vi "acqWaveform - 副本.vi"(0 "OSC in":refnum<visa-resource-name>, 1 "Points":u32=2000 max=7000, 2 "error in (no error)":errorcluster) -> (3 "OSC out":refnum<visa-resource-name>, 4 "time sequence":dbl[](array[numeric]), 5 "Voltage sequence":dbl[](array[numeric]), 6 "error out":errorcluster)   [LabVIEW 2016]
panel:
  out "XY Graph":cluster{dbl[], dbl[]}(graph)
  out "String":string
  in  "Channel":i8=1
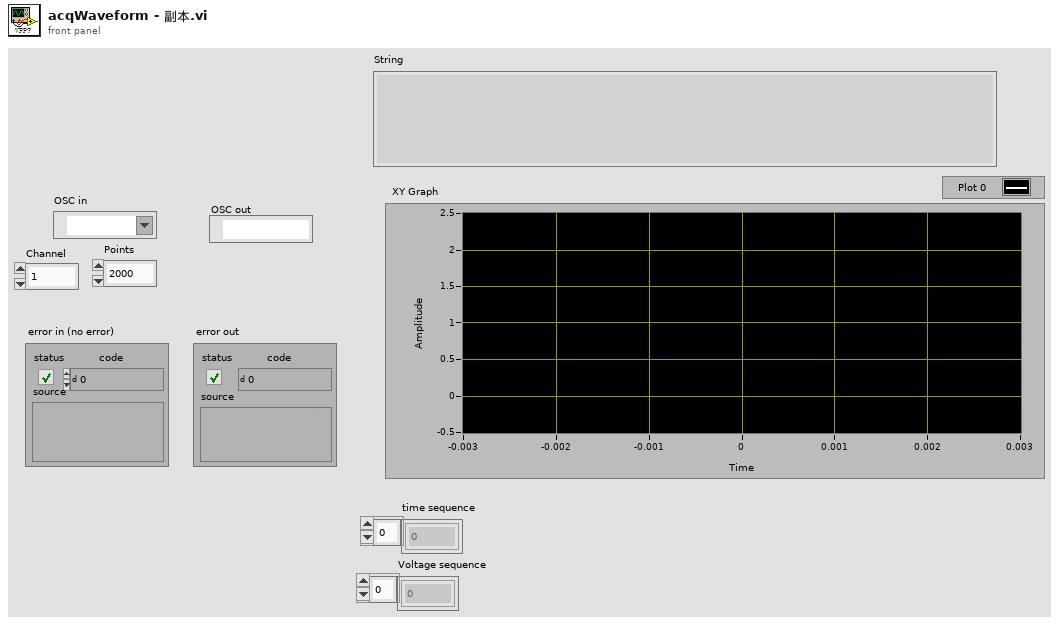
[diagram p1: front panel]
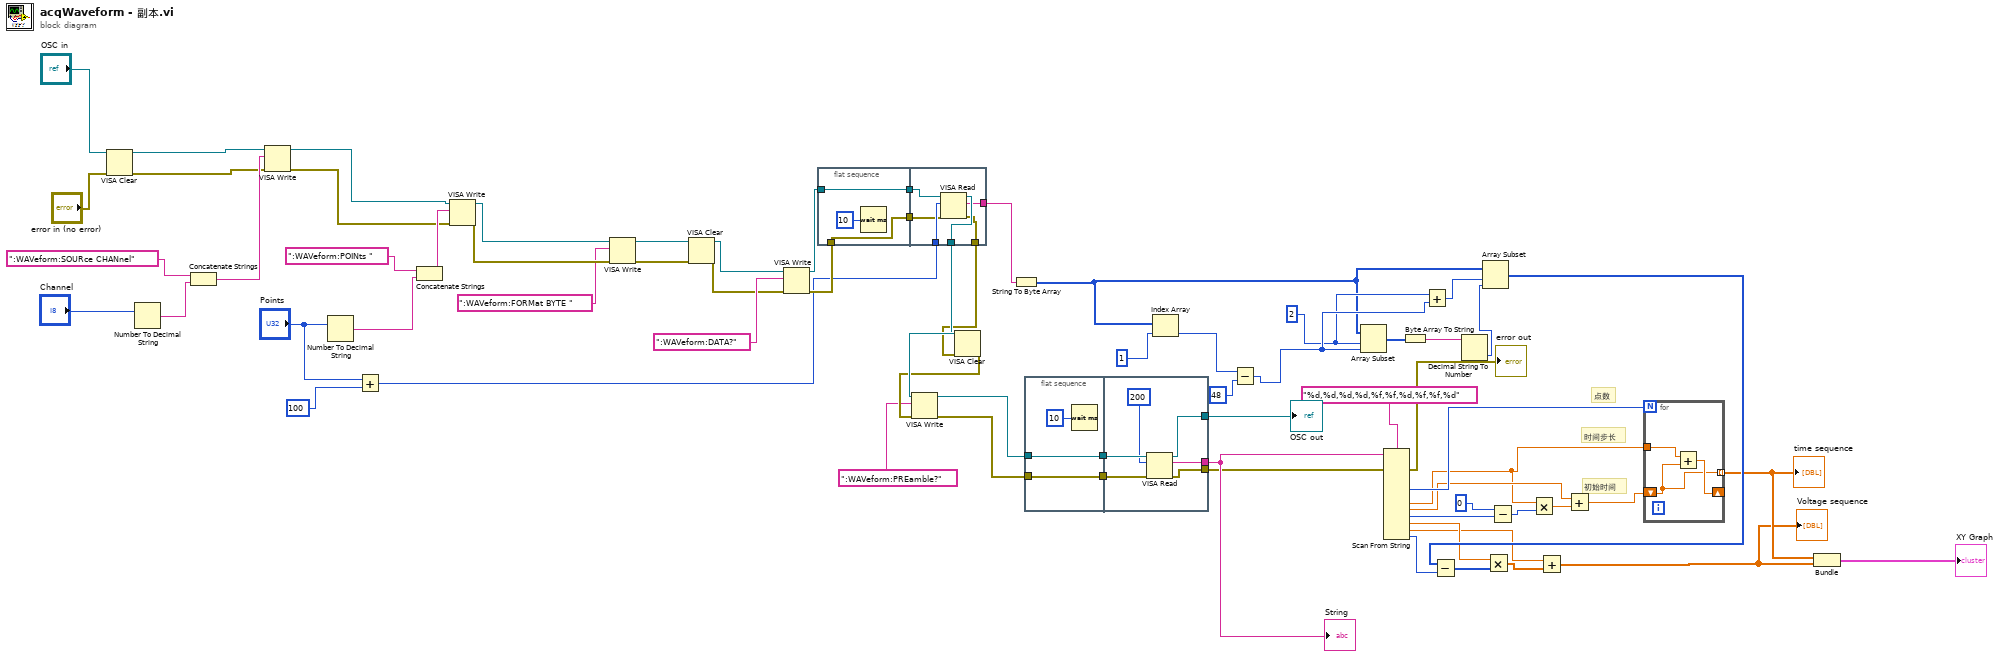
[diagram p0: block diagram]
diagram:
  w40 = 2
  # "初始时间"
  # "时间步长"
  # "点数"
  n1 = VISA Clear(VISA resource name="OSC in", error in (no error)="error in (no error)") -> (VISA resource name out=w63:refnum<visa-resource-name>, error out=w64:errorcluster)
  n2 = Number To Decimal String(number="Channel") -> (decimal integer string=w66:string)  [unwired: 1 in]
  n3 = Concatenate Strings(":WAVeform:SOURce CHANnel", w66) -> (w65:string)
  n4 = VISA Write(VISA resource name=w63, write buffer=w65, error in (no error)=w64) -> (VISA resource name out=w58:refnum<visa-resource-name>, error out=w59:errorcluster)  [unwired: 1 out]
  n5 = Number To Decimal String(number="Points") -> (decimal integer string=w62:string)  [unwired: 1 in]
  n6 = Add(x="Points", y=100) -> (x+y=w3:u32)
  n7 = Concatenate Strings(":WAVeform:POINts ", w62) -> (w60:string)
  n8 = VISA Write(VISA resource name=w58, write buffer=w60, error in (no error)=w59) -> (VISA resource name out=w57:refnum<visa-resource-name>, error out=w56:errorcluster)  [unwired: 1 out]
  n9 = VISA Write(VISA resource name=w57, write buffer=":WAVeform:FORMat BYTE ", error in (no error)=w56) -> (VISA resource name out=w54:refnum<visa-resource-name>, error out=w53:errorcluster)  [unwired: 1 out]
  n10 = VISA Clear(VISA resource name=w54, error in (no error)=w53) -> (VISA resource name out=w51:refnum<visa-resource-name>, error out=w50:errorcluster)
  n11 = VISA Write(VISA resource name=w51, write buffer=":WAVeform:DATA?", error in (no error)=w50) -> (VISA resource name out=w10:refnum<visa-resource-name>, error out=w8:errorcluster)  [unwired: 1 out]
  n12 = flat-sequence {
    tunnel: w10 -> [w72]
    tunnel: [w72] -> w9
    tunnel: w8 -> [w71]
    tunnel: [w71] -> w7
    tunnel: w9 -> [w74]
    tunnel: w7 -> [w75]
    tunnel: [w79] -> w6
    tunnel: [w78] -> w5
    tunnel: [w77] -> w4
    tunnel: w3 -> [w76]
    frame #0 {
      n13 = Wait (ms)(milliseconds to wait=u32 10) -> ()  [unwired: 1 out]
    }
    frame #1 {
      n14 = VISA Read(VISA resource name=w74, byte count=w76, error in (no error)=w75) -> (VISA resource name out=w79:refnum<visa-resource-name>, read buffer=w78:string, error out=w77:errorcluster)  [unwired: 1 out]
    }
  }
  n15 = VISA Clear(VISA resource name=w6, error in (no error)=w4) -> (VISA resource name out=w37:refnum<visa-resource-name>, error out=w36:errorcluster)
  n16 = VISA Write(VISA resource name=w37, write buffer=":WAVeform:PREamble?", error in (no error)=w36) -> (VISA resource name out=w34:refnum<visa-resource-name>, error out=w33:errorcluster)  [unwired: 1 out]
  n17 = String To Byte Array(string=w5) -> (unsigned byte array=w38:u8[])
  n18 = flat-sequence {
    tunnel: w33 -> [w81]
    tunnel: w34 -> [w82]
    tunnel: [w82] -> w2
    tunnel: [w81] -> w1
    tunnel: [w86] -> w32
    tunnel: [w84] -> w30
    tunnel: [w83] -> w29
    tunnel: w2 -> [w88]
    tunnel: w1 -> [w87]
    frame #0 {
      n19 = Wait (ms)(milliseconds to wait=u32 10) -> ()  [unwired: 1 out]
    }
    frame #1 {
      n20 = VISA Read(VISA resource name=w88, byte count=200, error in (no error)=w87) -> (VISA resource name out=w86:refnum<visa-resource-name>, read buffer=w84:string, error out=w83:errorcluster)  [unwired: 1 out]
    }
  }
  n21 = Index Array(array=w38, index=1) -> (element=w46:u8)
  n22 = Subtract(x=w46, y=48) -> (x-y=w41:i32)
  n23 = Array Subset(array=w38, index=w40, length=w41) -> (w44:u8[])
  n24 = Scan From String(format string="%d,%d,%d,%d,%f,%f,%d,%f,%f,%d", input string=w30, error in=w29) -> (error out=→"error out":errorcluster, output 3=w27:i32, output 5=w20:dbl, output 6=w22:dbl, output 7=w26:i32, output 8=w16:dbl, output 9=w15:dbl, output 10=w18:i32)  [unwired: 14 in, 2 out]
  n25 = Byte Array To String(unsigned byte array=w44) -> (string=w43:string)
  n26 = Add(x=w40, y=w41) -> (x+y=w39:i32)
  n27 = Decimal String To Number(string=w43) -> (number=w42:i32)  [unwired: 2 in, 1 out]
  n28 = Array Subset(array=w38, index=w39, length=w42) -> (w19:u8[])
  n29 = Subtract(x=w19, y=w18) -> (x-y=w17:i32[])
  n30 = Multiply(x=w16, y=w17) -> (x*y=w14:dbl[])
  n31 = Subtract(x=0, y=w26) -> (x-y=w24:i32)
  n32 = Multiply(x=w20, y=w24) -> (x*y=w23:dbl)
  n33 = Add(x=w15, y=w14) -> (x+y=w11:dbl[])
  "Voltage sequence" <- w11
  n34 = Add(x=w22, y=w23) -> (x+y=w21:dbl)
  n35 = for {
    N: w27 -> [_]
    shift-right: [w91] -> _
    shift-left: w21 -> [w89]
    tunnel: w20 -> [w90]
    tunnel: [w89] -> w13 mode=indexing
    n36 = Add(x=w90, y=w89) -> (x+y=w91:dbl)
  }
  "time sequence" <- w13
  n37 = Bundle(w13, w11) -> (→"XY Graph":cluster{dbl[], dbl[]})  [unwired: 1 in]
  "OSC out" <- w32
  "String" <- w30
